vi "initialize.vi"(0 "Port":T1 {"North" format="%#_10f"; "East" format="%#_8f"}, 1 "Starboard":T1 {"North" format="%#_10f"; "East" format="%#_8f"}, 2 "Tolerance (m)":dbl, 3 "Error In":errorcluster) -> (5 "PassBouy.lvclass out":refnum<class "PassBouy.lvclass">, 6 "Error Out":errorcluster)   [LabVIEW 2012, in "PassBouy.lvclass"]
doc: "Creates a \"PassBouys\" mission. Given two bouy locations (Port and Starboard), the mission will calculate the waypoints nessisary to guide the boat through the two bouys"
uses:
  PassBouy.lvclass
  Data/TypeDefs/MissionTypeControl.ctl
  Data/TypeDefs/UTM Location.ctl
panel:
  in  "PassBouy.lvclass":refnum<class "PassBouy.lvclass">
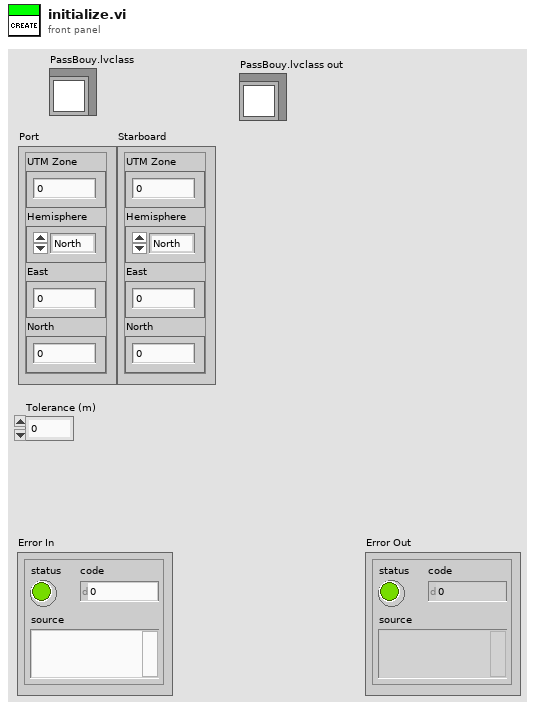
[diagram p1: front panel]
types:
  T1 = typedef "UTM Location.ctl" = cluster{"UTM Zone":dbl, "Hemisphere":enum16{"North", "South"}, "East":dbl, "North":dbl}
  T2 = typedef "MissionTypeControl.ctl" = enum16{"Idle at Point", "Drive to Waypoint", "Round Buoy to Port", "Round Buoy to Starboard", "Pass Between Buoys", "Station Keeping"}
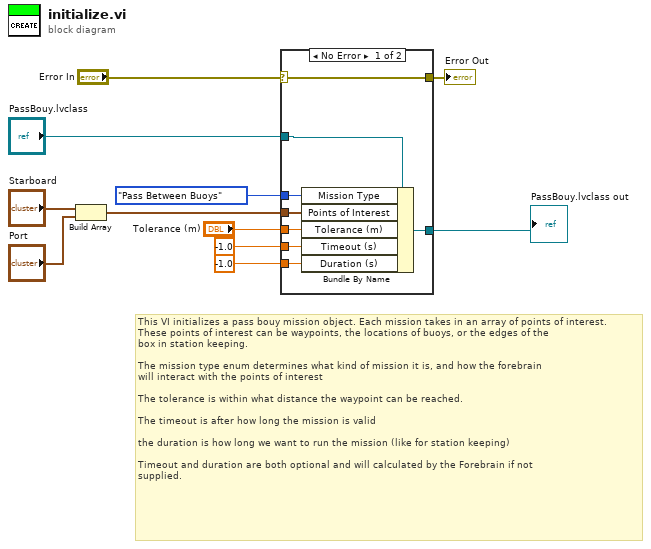
[diagram p0: block diagram]
diagram:
  # "This VI initializes a pass bouy mission object. Each mission takes in an array of points of interest.\nThese points of interest can be waypoints, the locations of buoys, or the edges of the \nbox in station keeping. \n\nThe mission type enum determines what kind of mission it is, and how the forebrain \nwill interact with the points of interest\n\nThe tolerance is within what distance the waypoint can be reached. \n\nThe timeout is after how long the mission is valid\n\nthe duration is how long we want to run the mission (like for station keeping)\n\nTimeout and duration are both optional and will calculated by the Forebrain if not \nsupplied."
  n1 = Build Array("Starboard", "Port") -> (w1:T1[])
  n2 = case shown="No Error" "Error In" {
    selector: "Error In" -> [w19 w20]
    tunnel: [w19 w20] -> w10
    tunnel: MissionTypeControl."Pass Between Buoys" ("Mission Type") -> [w18 _]
    tunnel: "Tolerance (m)" -> [w17 _]
    tunnel: -1.0 ("Timeout (s)") -> [w16 _]
    tunnel: -1.0 ("Duration (s)") -> [w15 _]
    tunnel: "PassBouy.lvclass" -> [w14 w21]
    tunnel: [w13 w21] -> w5
    tunnel: w1 -> [w12 _]
    frame No Error {
      n3 = Bundle By Name(cluster=w14, "Mission Type"=w18, "Points of Interest"=w12, "Tolerance (m)"=w17, "Timeout (s)"=w16, "Duration (s)"=w15) -> (w13:refnum<class "PassBouy.lvclass">)
    }
    frame Error {
    }
  }
  "Error Out" <- w10
  "PassBouy.lvclass out" <- w5
